vi "CreateCSVColumnHeaders.vi"() -> (3 "Column Headers":string)   [LabVIEW 2012]
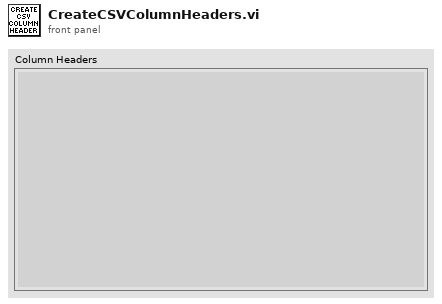
[diagram p1: front panel]
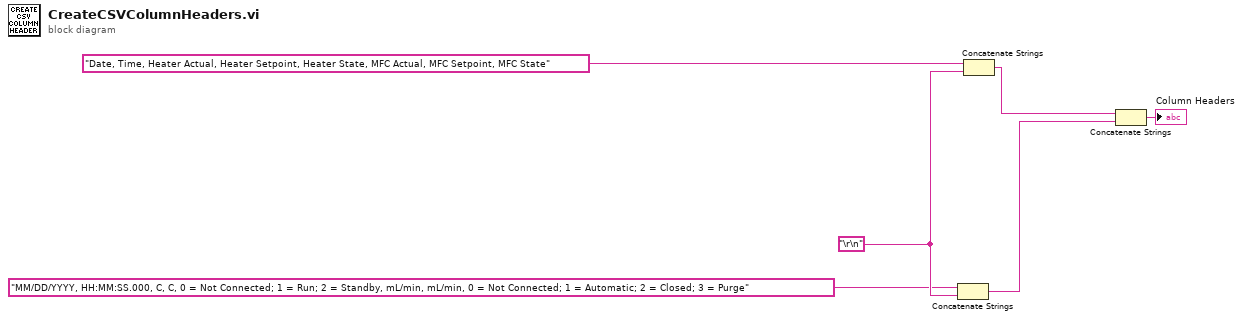
[diagram p0: block diagram]
diagram:
  w2 = "\r\n"
  n1 = Concatenate Strings("MM/DD/YYYY, HH:MM:SS.000, C, C, 0 = Not Connected; 1 = Run; 2 = Standby, mL/min, mL/min, 0 = Not Connected; 1 = Automatic; 2 = Closed; 3 = Purge", w2) -> (w4:string)
  n2 = Concatenate Strings("Date, Time, Heater Actual, Heater Setpoint, Heater State, MFC Actual, MFC Setpoint, MFC State", w2) -> (w5:string)
  n3 = Concatenate Strings(w5, w4) -> (→"Column Headers":string)
